vi "poly_asynch_wait_notify.vi"(8 "error in":errorcluster, 10 "asynch wait ref in":T1) -> (0 "error out":errorcluster)   [LabVIEW 2015, in "_timing_tools_polys.lvlib"]
uses:
  _timing_tools_polys.lvlib
  asynch_wait_ref.ctl
  boolean_notifier.ctl
  poly_timing_tools_eco_plus.vi
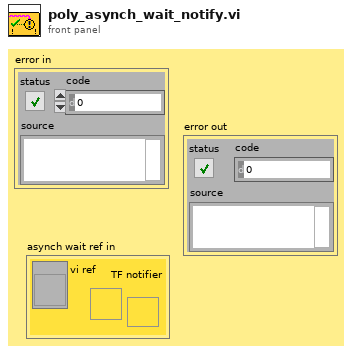
[diagram p1: front panel]
types:
  T1 = typedef "_timing_tools_polys.lvlib/asynch_wait_ref.ctl" = cluster{"vi ref":refnum<vi>, "TF notifier":T2}
  T2 = typedef "_timing_tools_polys.lvlib/boolean_notifier.ctl" = refnum<notifier>
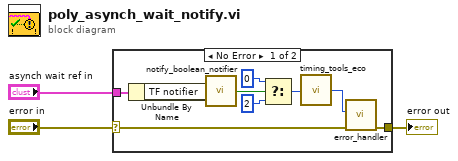
[diagram p0: block diagram]
diagram:
  n1 = case shown="No Error" "error in" {
    selector: "error in" -> [w7 w13]
    tunnel: [w6 w13] -> w3
    tunnel: "asynch wait ref in" -> [w12 _]
    frame No Error {
      n2 = Unbundle By Name(w12) -> ("TF notifier"=w11:T2)
      n3 = call "notify_boolean_notifier.vi"("TF notifier"=w11) -> ("notified?"=w10:bool)  [unwired: 8 in]
      n4 = Select(t=0 ("code (0 = no error)"), s=w10, f=2) -> (s? t:f=w5:i32)
      n5 = call-poly "timing_tools_eco.vi"("code (w/out eco)"=w5) -> ("code (+ eco)"=w4:i32)  [unwired: 4 in]
      n6 = call "error_handler.vi"("error in (no error)"=w7, "code (0 = no error)"=w4) -> ("error out"=w6:errorcluster)  [unwired: 8 in, 1 out]
    }
    frame Error {
    }
  }
  "error out" <- w3
